vi "GetBars.vi"(8 "error in (no error)":errorcluster, 10 "Munged Input":string, 11 "BarCode in":refnum<class "BarCode.lvclass">) -> (0 "error out":errorcluster, 2 "BarWidths":T1[][](array[typedef]), 3 "BarCode out":refnum<class "BarCode.lvclass">)   [LabVIEW 2013, in "BarCodes.lvlib" / "BarCode.lvclass"]
doc: "Gets the bars of the bar code. The bars are specified as an array of bar widths from left to right. This must be overridden by classes extending BarCode.lvclass."
uses:
  BarCode.lvclass
  Bar.ctl
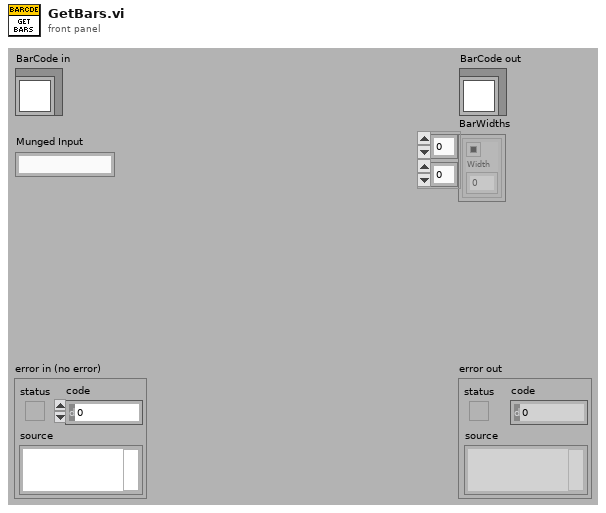
[diagram p1: front panel]
types:
  T1 = typedef "BarCodes.lvlib/BarCode.lvclass/Bar.ctl" = cluster{"Color":u32, "Width":u8}
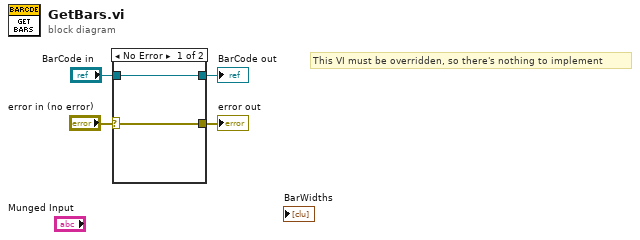
[diagram p0: block diagram]
diagram:
  # "This VI must be overridden, so there's nothing to implement"
  n1 = case shown="No Error" "error in (no error)" {
    selector: "error in (no error)" -> [w5 w8]
    tunnel: [w5 w8] -> w3
    tunnel: [w6 w7] -> w1
    tunnel: "BarCode in" -> [w6 w7]
    frame No Error {
    }
    frame Error {
    }
  }
  "error out" <- w3
  "BarCode out" <- w1
